vi "Mark Phonation Cutoff (Incomplete).vi"(7 "Error In":errorcluster, 8 "File Path":path, 10 "Pressure/Audio":dynamicdata(graph)) -> (0 "Error Out":errorcluster, 1 "File Path Indicator":path, 2 "Interruption Time":dbl, 3 "Cutoff Pressure":dbl)   [LabVIEW 2020, in "AnalysisSupport.lvlib"]
uses:
  AnalysisSupport.lvlib
  <vilib>/Waveform/WDTOps.llb/WDT Get XY Value DBL.vi
panel:
  in  "Done":bool
  out "Enlarged":dynamicdata(graph)
  out "Pressure/Audio":dynamicdata(graph)
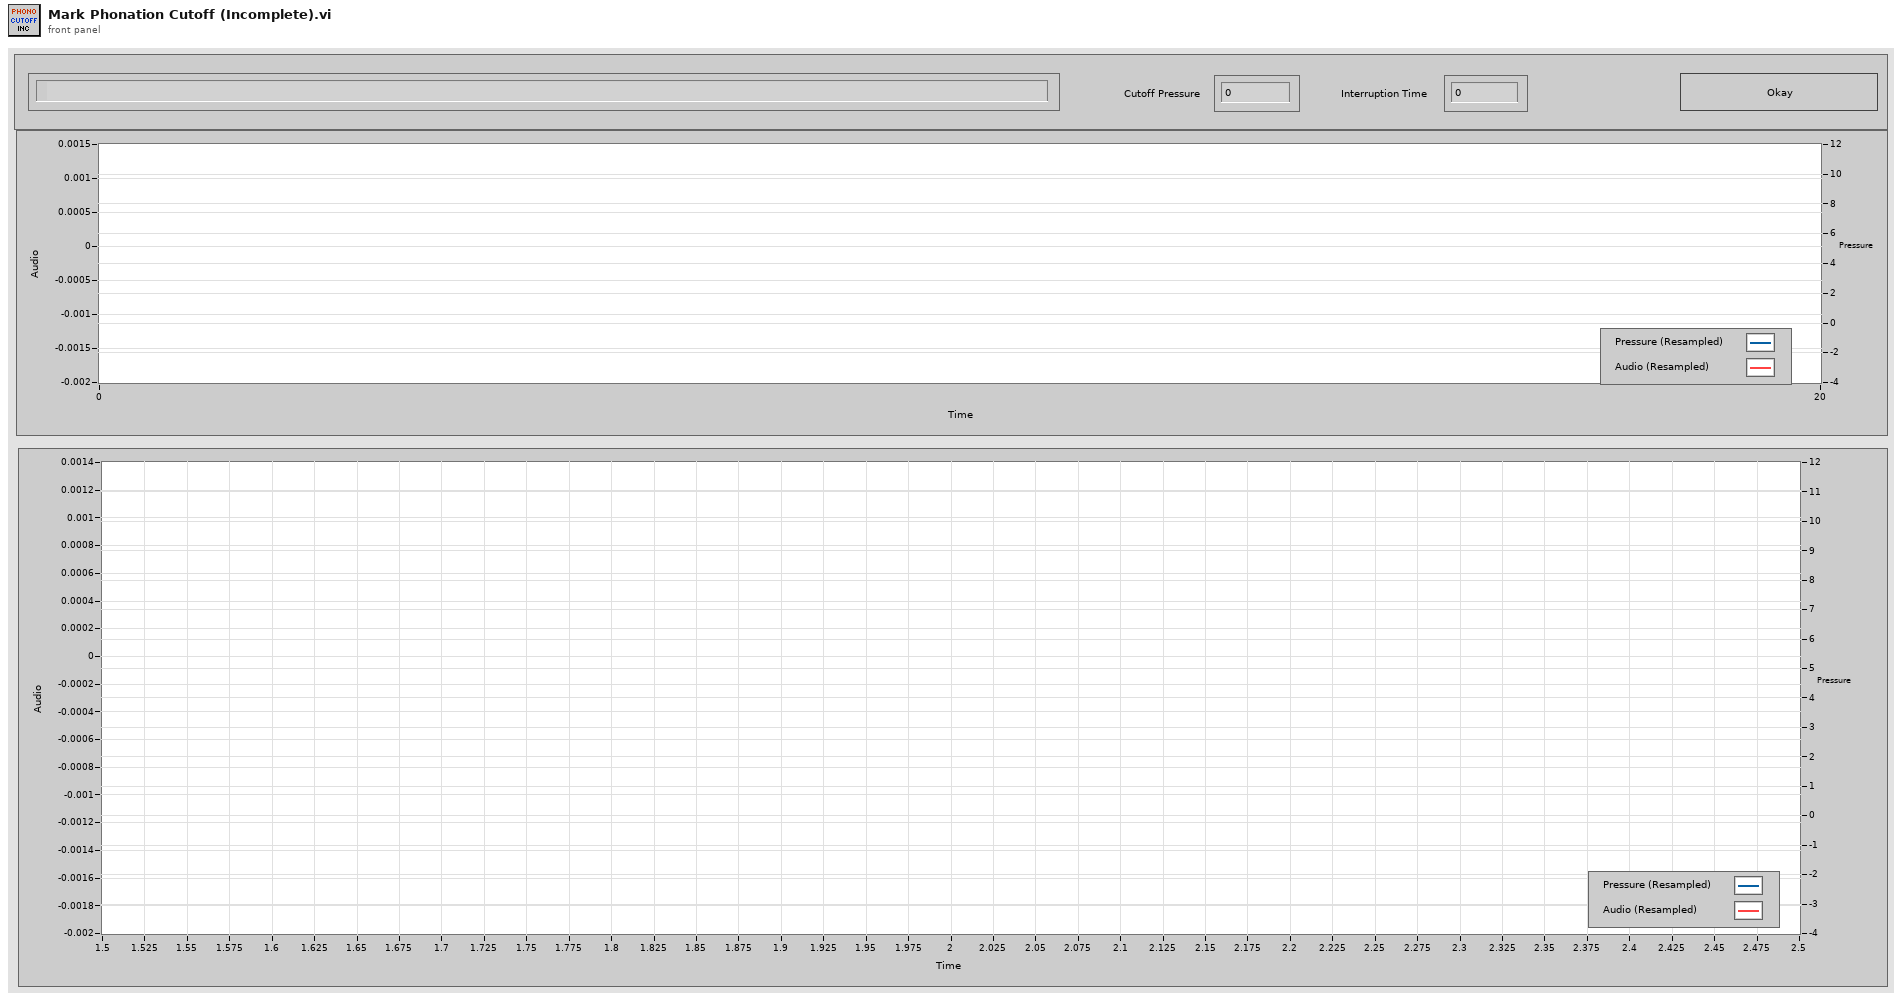
[diagram p1: front panel]
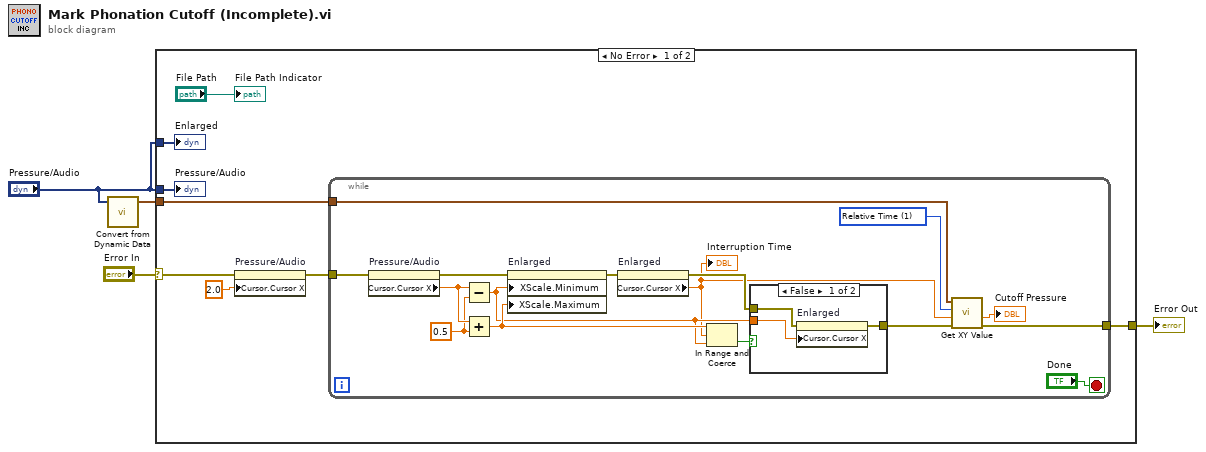
[diagram p0: block diagram]
diagram:
  n1 = call "Convert from Dynamic Data"("Dynamic Data Type"="Pressure/Audio") -> ("Waveform"=w2:waveform(dbl))  [unwired: 3 in]
  n2 = case shown="No Error" "Error In" {
    selector: "Error In" -> [w5 w33]
    tunnel: [w6 w33] -> w4
    tunnel: "Pressure/Audio" -> [w7 _]
    tunnel: "Pressure/Audio" -> [w9 _]
    tunnel: w2 -> [w8 _]
    frame No Error {
      n3 = property on="Pressure/Audio" class="WFGraph (strict)"(error in=w5, "Cursor.Cursor X"=2.0 ("Cursor.Cursor Position:Cursor X")) -> (error out=w10:errorcluster)  [unwired: 1 in, 1 out]
      n4 = while {
        tunnel: w10 -> [w28]
        tunnel: w8 -> [w27]
        tunnel: [w13] -> w6
        stop <- "Done" stop-if-true
        w17 = u16 1 items=["Samples", "Relative Time"] ("Y position format")
        w24 = 0.5 ("y")
        n5 = property on="Pressure/Audio" class="WFGraph (strict)"(error in=w28) -> (error out=w22:errorcluster, "Cursor.Cursor X"=w25:dbl)  [unwired: 1 in, 1 out]
        n6 = Subtract(x=w25, y=w24) -> (x-y=w18:dbl)
        n7 = Add(x=w25, y=w24) -> (x+y=w23:dbl)
        n8 = property on="Enlarged" class="WFGraph (strict)"(error in=w22, "XScale.Minimum"=w18, "XScale.Maximum"=w23) -> (error out=w21:errorcluster)  [unwired: 1 in, 1 out]
        n9 = property on="Enlarged" class="WFGraph (strict)"(error in=w21) -> (error out=w20:errorcluster, "Cursor.Cursor X"=w16:dbl)  [unwired: 1 in, 1 out]
        "Interruption Time" <- w16
        n10 = In Range and Coerce(upper limit=w23, x=w16, lower limit=w18) -> (In Range?=w26:bool)  [unwired: 1 out]
        n11 = case shown="False" w26 {
          tunnel: w20 -> [w31 w32]
          tunnel: [w30 w32] -> w19
          tunnel: w18 -> [w29 _]
          frame False {
            n12 = property on="Enlarged" class="WFGraph (strict)"(error in=w31, "Cursor.Cursor X"=w29) -> (error out=w30:errorcluster)  [unwired: 1 in, 1 out]
          }
          frame True {
          }
        }
        n13 = call-poly <vilib>:"Get XY Value.vi"("error in (no error)"=w19, "Y position"=w16, "Y position format"=w17, "waveform in"=w27) -> ("error out"=w13:errorcluster, "Y value"=→"Cutoff Pressure":dbl)  [unwired: 3 in, 3 out]
      }
      "File Path Indicator" <- "File Path"
      "Enlarged" <- w9
      "Pressure/Audio" <- w7
    }
    frame Error {
    }
  }
  "Error Out" <- w4
